vi "genIOL_Injection2.vi"(4 "Initial guess":dbl[](array[numeric])=[-67.99974822998047, 12.682350158691406, -0.8997803330421448, -0.012297453358769417], 6 "DH Params":cluster{"d_DH":dbl[][], "ty":dbl[][]}, 7 "endJ5":dbl=3200.0, 8 "OCT offset":dbl=11.0, 9 "endPt":dbl[](array[numeric])=[8.48840241312517, 12.608494085712664, 1.4642729158965477], 10 "PC path":path=path "D:/IRISSoft LV2016 beta/Host Demo/ThorlabsData/Eye1/VSCAN_0008.raw", 11 "Iris path":path=path "D:/IRISSoft LV2016 beta/Host Demo/ThorlabsData/Eye1/VSCAN_0007.raw") -> (0 "Whole_traj":dbl[][](array[numeric]), 1 "Inject_traj":dbl[][](array[numeric]))   [LabVIEW 2016]
uses:
  <vilib>/Math Plots/3D Math Plots/3D Scatter/3D Scatter XCtrl/3D Scatter.xctl
  <vilib>/Utility/file.llb/Read Delimited Spreadsheet (DBL).vi
  <vilib>/Utility/file.llb/Write Delimited Spreadsheet (DBL).vi
  <vilib>/Math Plots/3D Math Plots/3D Scatter/3D Scatter Datatype/Public/Plot Helper (Vector).vi
  <vilib>/Analysis/NI_AALBase.lvlib
  <vilib>/Analysis/1siggen.llb/Ramp Pattern by Samples.vi
  <vilib>/gmath/NI_Gmath.lvlib
  Subsystems/Global Variables.vi
  <vilib>/Math Plots/3D Math Plots/3D Scatter/3D Scatter Datatype/3D Scatter Datatype.lvclass
  <vilib>/Math Plots/3D Math Plots/3D Plot/3D Plot Datatype/3D Plot Datatype.lvclass
panel:
  in  "Theta":dbl
  out "Actual Injection Plot 2":refnum<class "3D Plot Datatype.lvclass">[](xcontrol)
  out "current loop # 2":dbl
  out "Actual joint angles":dbl[][](array[numeric])
  out "Planned joint angles":dbl[][](array[numeric])
  out "Planned injection":dbl[][](array[numeric])
  out "time":dbl[](array[numeric])
  out "Implement joint angles":dbl[][](graph)
  out "min dist":dbl
  out "Planed joint angles":dbl[][](graph)
  out "Actual joint angles":dbl[][](graph)
  out "traj":dbl[][](array[numeric])
  out "max dist":dbl
  out "Offset":dbl[][](array[numeric])
  out "Planed Injection Plot":refnum<class "3D Plot Datatype.lvclass">[](xcontrol)
  out "current loop #":dbl
  out "x coordinates size 3":dbl
  out "x coordinates size 2":dbl
  out "x coordinates size":dbl
  out "x coordinates":dbl[](array[numeric])
  out "z coordinates":dbl[](array[numeric]) format="%#_13g"
  out "y coordinates":dbl[](array[numeric]) format="%#_13g"
  out "x coodi 2nd":dbl[](array[numeric]) format="%#_13g"
  in  "Total Time":dbl=60.0
  in  "Arm ID Ind":i32
  in  "Tip out Posit":dbl[](array[numeric])=[0.0, 0.0, 0.0] caption="Position [mm]" format="%#.3f"
  out "zVisTraj":dbl[](array[numeric]) format="%_6g"
  out "yVisTraj":dbl[](array[numeric]) format="%_6g"
  out "xVisTraj":dbl[](array[numeric]) format="%_6g"
  in  "Sampling Rate [Hz]":i32=1000
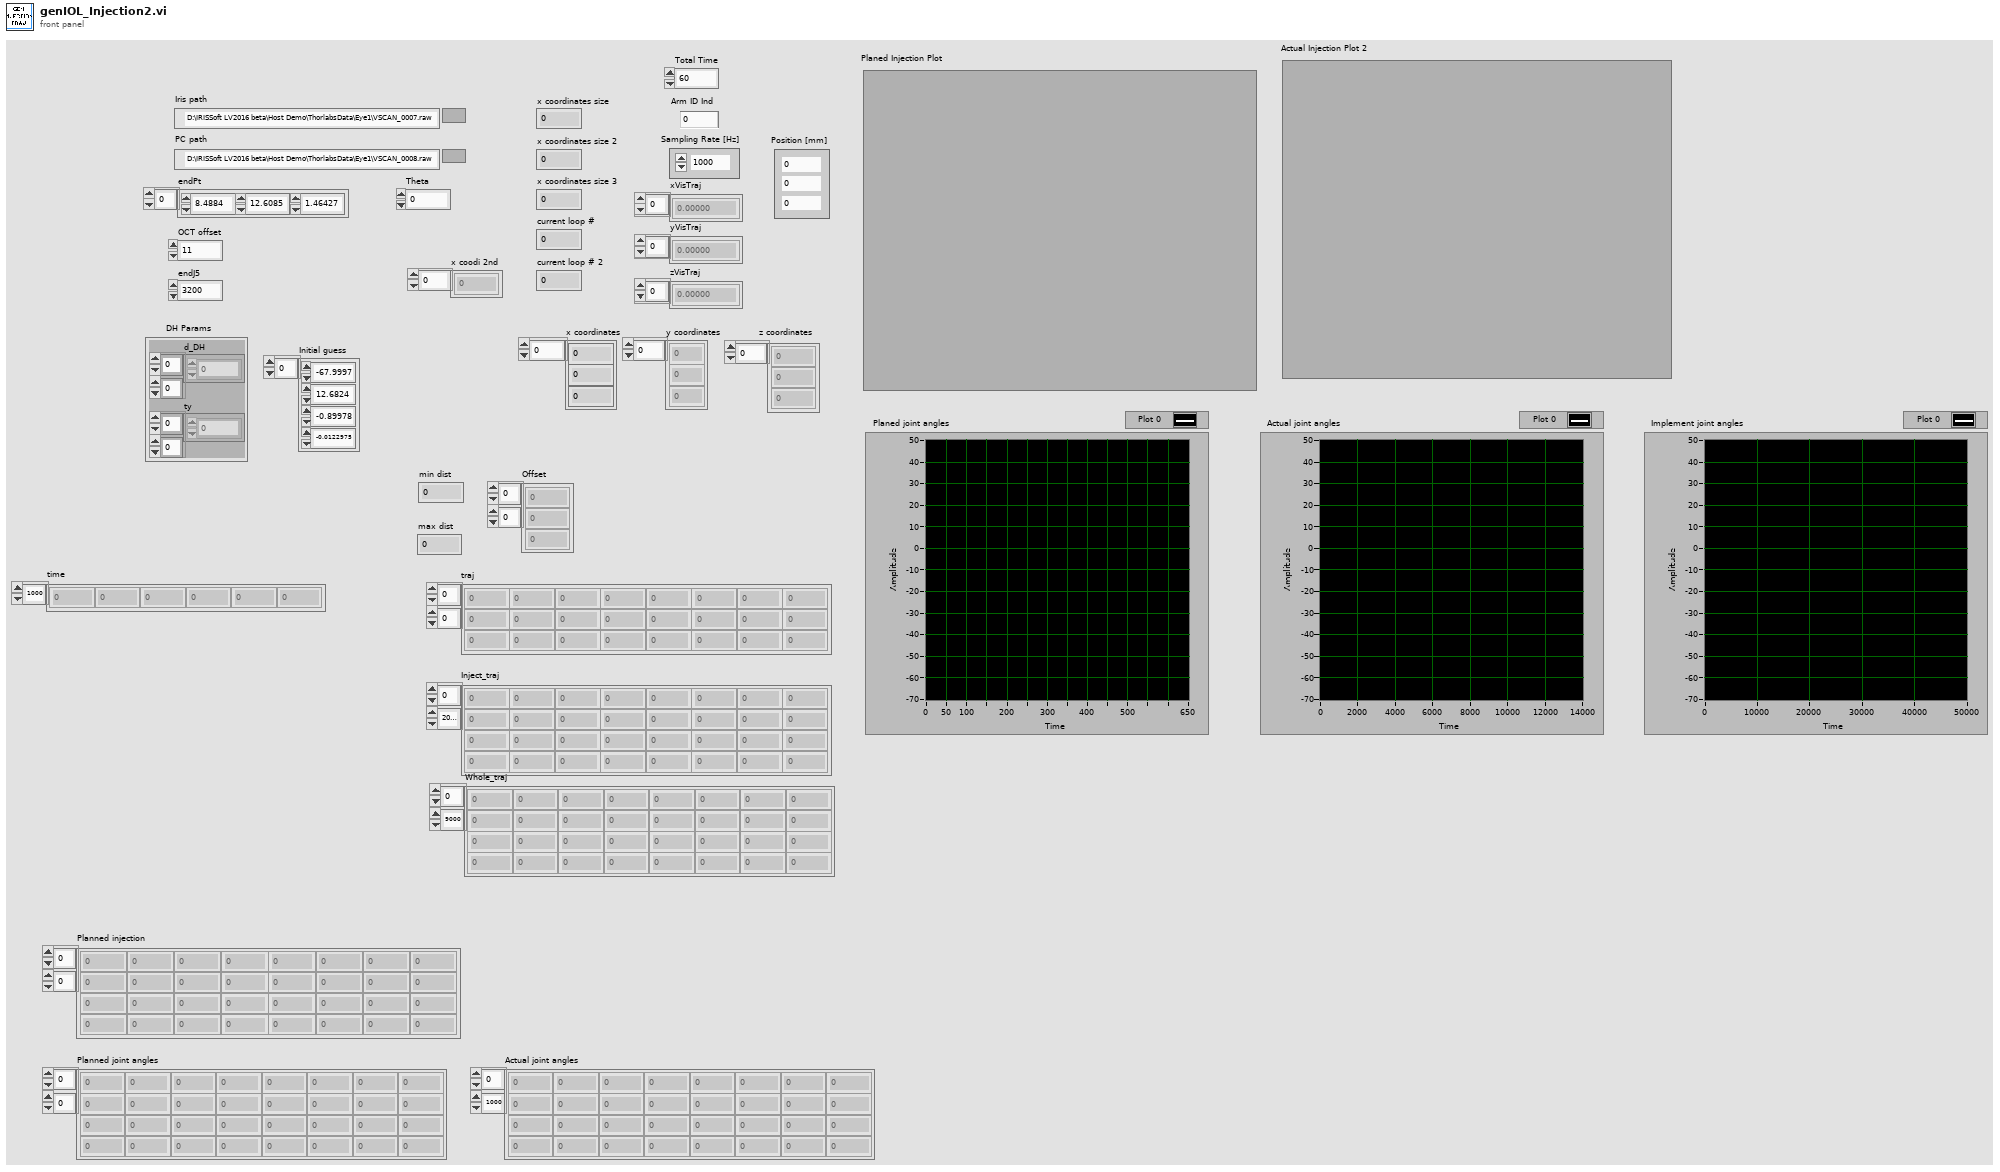
[diagram p1: front panel]
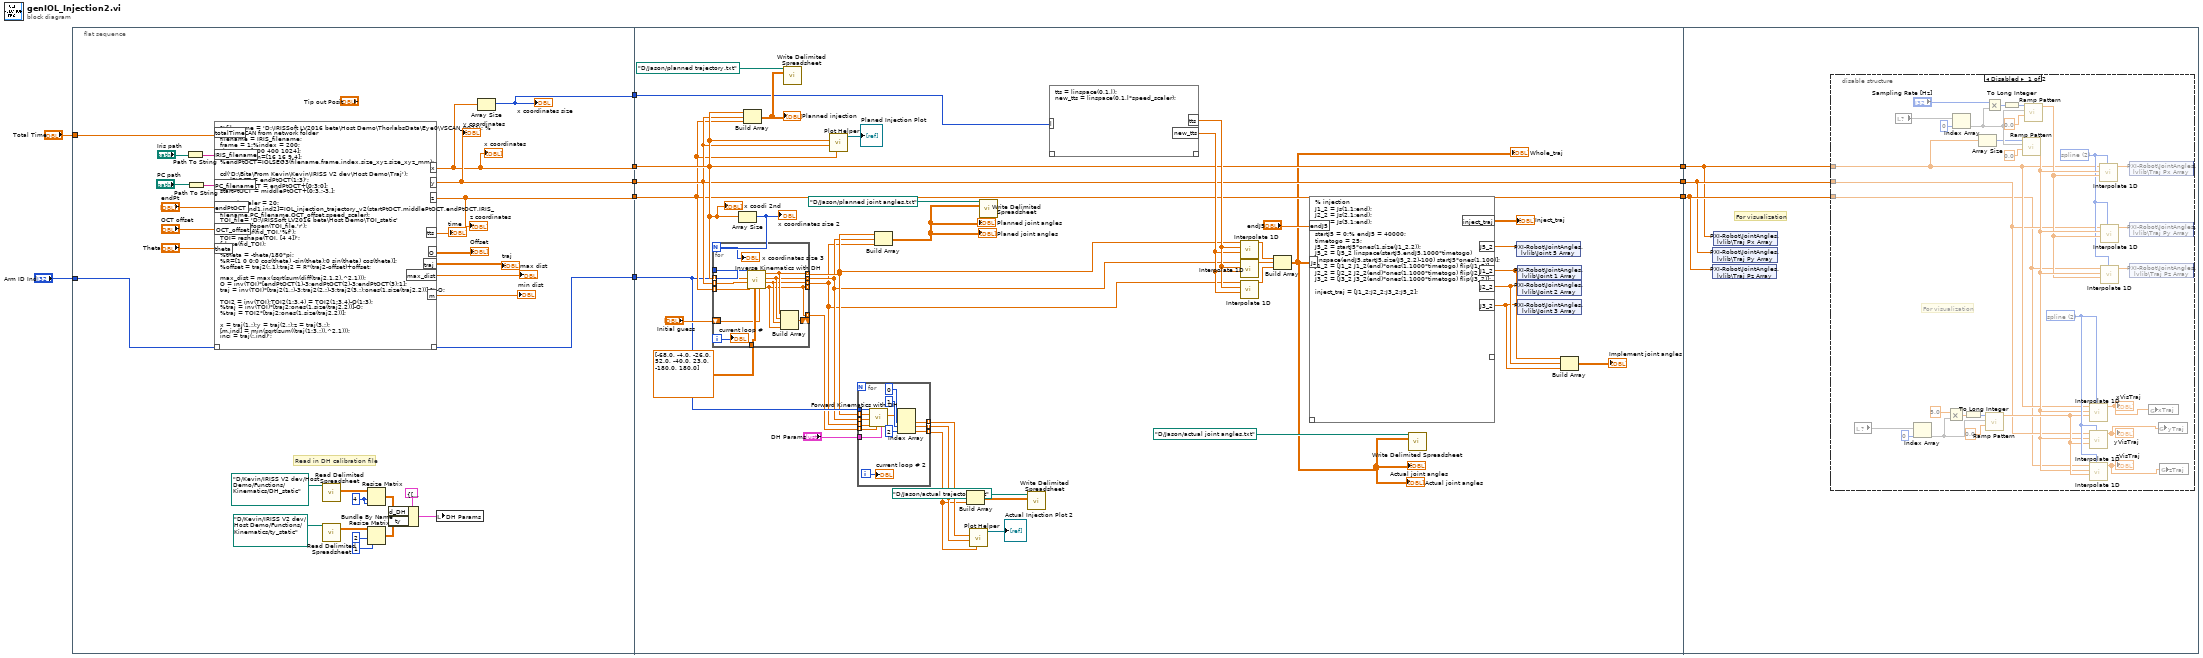
[diagram p0: block diagram]
diagram:
  n1 = flat-sequence {
    tunnel: "Arm ID Ind" -> [w12]
    tunnel: [w36] -> w6
    tunnel: [w38] -> w5
    tunnel: [w37] -> w4
    tunnel: "Total Time" -> [w39]
    tunnel: [w24] -> w2
    tunnel: [w12] -> w1
    tunnel: [w62] -> w9
    tunnel: [w61] -> w8
    tunnel: [w60] -> w7
    tunnel: w6 -> [w62]
    tunnel: w5 -> [w61]
    tunnel: w4 -> [w60]
    tunnel: w2 -> [w43]
    tunnel: w1 -> [w54]
    tunnel: w9 -> [w105]
    tunnel: w8 -> [w106]
    tunnel: w7 -> [w107]
    frame #0 {
      w21 = 4 ("number of rows")
      # "Read in DH calibration file"
      n2 = Path To String(path="Iris path") -> (string=w31:string)
      n3 = Path To String(path="PC path") -> (string=w32:string)
      n4 = script code="%filename = 'D:\\IRISSoft LV2016 beta\\Host Demo\\ThorlabsData\\Eye0\\VSCAN_0021'; % read VSCAN from network folder \nfilename = IRIS_filename;\nframe = 1;%index = 200;\nsize_xyz=[400 400 1024];\nsize_xyz_mm=[16 16 9.4];\n%endPtOCT=IOLSEG3(filename,frame,index,size_xyz,size_xyz_mm);\n\ncd('D:\\Bita\\From Kevin\\Kevin\\IRISS V2 dev\\Host Demo\\Traj');\nendPtOCT = endPtOCT(1:3)';\nmiddlePtOCT = endPtOCT+[0;3;0];\nstartPtOCT = middlePtOCT+[0;3.;-3.];\n\nspeed_scaler = 20;\n[tts,traj2,ind1,ind2]=IOL_injection_trajectory_v2(startPtOCT,middlePtOCT,endPtOCT,IRIS_filename,PC_filename,OCT_offset,speed_scaler);\nTOI_file= 'D:\\IRISSoft LV2016 beta\\Host Demo\\TOI_static'\nfid_TOI = fopen(TOI_file,'r');\nTOI=fscanf(fid_TOI,'%f');\nTOI= reshape(TOI, [4 4])';\nfclose(fid_TOI);\n\n%theta = -theta/180*pi;\n%R=[1 0 0;0 cos(theta) -sin(theta);0 sin(theta) cos(theta)];\n%offset = traj2(:,1);traj2 = R*(traj2-offset)+offset;\n\nmax_dist = max(sqrt(sum(diff(traj2,1,2).^2,1)));\nO = inv(TOI)*[endPtOCT(1)-3;endPtOCT(2)-3;endPtOCT(3);1];\ntraj = inv(TOI)*[traj2(1,:)-3;traj2(2,:)-3;traj2(3,:);ones(1,size(traj2,2))];%-O;\n\nTOI2 = inv(TOI);TOI2(1:3,4) = TOI2(1:3,4)-O(1:3);\n%traj = inv(TOI)*[traj2;ones(1,size(traj2,2))]-O;\n%traj = TOI2*[traj2;ones(1,size(traj2,2))];\n\nx = traj(1,:);y = traj(2,:);z = traj(3,:);\n[m,ind] = min(sqrt(sum((traj(1:3,:)).^2,1)));\ninci = traj(:,ind)';"("totalTime"=w39, "IRIS_filename"=w31, "PC_filename"=w32, "endPtOCT"="endPt", "OCT_offset"="OCT offset", "theta"="Theta") -> ("x"=w36:dbl[], "y"=w38:dbl[], "z"=w37:dbl[], "O"=→"Offset":dbl[][], "max_dist"=→"max dist":dbl, "traj"=→"traj":dbl[][], "m"=→"min dist":dbl, "tts"=→"time":dbl[])  [unwired: 1 in, 1 out]
      "y coordinates" <- w38
      "z coordinates" <- w37
      "x coordinates" <- w36
      n5 = call-poly <vilib>:"Read Delimited Spreadsheet.vi"("file path (dialog if empty)"=path "D:/Kevin/IRISS V2 dev/Host Demo/Functions/Kinematics/DH_static" ("file path (use dialog)")) -> ("all rows"=w22:dbl[][])  [unwired: 9 in, 5 out]
      n6 = call-poly <vilib>:"Read Delimited Spreadsheet.vi"("file path (dialog if empty)"=path "D:/Kevin/IRISS V2 dev/Host Demo/Functions/Kinematics/ty_static" ("file path (use dialog)")) -> ("all rows"=w20:dbl[][])  [unwired: 9 in, 5 out]
      n7 = Resize Matrix(1:w21, 2:w21, 4:w22) -> (0:w16:dbl[][])
      n8 = Resize Matrix(1:1 ("number of columns"), 2:2 ("number of rows"), 4:w20) -> (0:w15:dbl[][])
      n9 = Bundle By Name(cluster=cluster{"d_DH":dbl[][], "ty":dbl[][]} {"d_DH"=[[0.0, -0.04858099004841317, 1.1971672750675049, 0.0], [0.0, -1.576475511297109, 0.0, 0.0], [-0.3552491783526254, 0.0, -1.1064589410656984, 0.2058446720735121], [-1.0573457532495087, 1.0278049025155533, 0.011917110633363169, -0.004023577880993236]], "ty"=[[0.04320445582455471], [0.011728642746432275]]} ("input cluster"), "d_DH"=w16, "ty"=w15) -> (w13:cluster{"d_DH":dbl[][], "ty":dbl[][]})
      n10 = local write "DH Params"(w13) -> ()
      n11 = Array Size(array=w36) -> (size(s)=w24:i32)
      "x coordinates size" <- w24
    }
    frame #1 {
      n12 = Array Size(array=w62) -> (size(s)=w77:i32)
      "x coordinates size 2" <- w77
      n13 = for {
        N: w77 -> [w104]
        tunnel: w54 -> [w101]
        tunnel: w62 -> [w100] mode=indexing
        tunnel: w61 -> [w99] mode=indexing
        tunnel: w60 -> [w98] mode=indexing
        tunnel: [w94] -> w47 mode=indexing
        tunnel: [w95] -> w48 mode=indexing
        tunnel: [w93] -> w46 mode=indexing
        tunnel: dbl[][] [[-68.0, -4.0], [-26.0, 52.0], [-40.0, 23.0], [-180.0, 180.0]] ("Joint Limits") -> [w97]
        shift-right: [w102] -> _
        shift-left: "Initial guess" -> [w96]
        tunnel: [w92] -> _ mode=indexing
        tunnel: [w92] -> w40 mode=indexing
        i -> [w103]
        n14 = call "Inverse Kinematics with DH.vi"("Initial guess"=w96, "Joint Limits"=w97, "armID"=w101, "z"=w98, "y"=w99, "x"=w100) -> ("j4"=w92:dbl, "j3"=w93:dbl, "j2"=w94:dbl, "j1"=w95:dbl)  [unwired: 2 in]
        n15 = Build Array(w95, w94, w93, w92) -> (w102:dbl[])
        "x coordinates size 3" <- w104
        "current loop #" <- w103
      }
      n16 = Build Array(w62, w61, w60) -> (w59:dbl[][])
      "Planned injection" <- w59
      n17 = call-poly <vilib>:"Write Delimited Spreadsheet.vi"("file path (dialog if empty)"=path "D:/Jason/planned trajectory.txt", "2D data"=w59) -> ()  [unwired: 12 in, 2 out]
      n18 = call-poly <vilib>:"Plot Helper.vi"("z vector"=w60, "y vector"=w61, "x vector"=w62) -> ("3D Plot lvclass Array out"=→"Planed Injection Plot":refnum<class "3D Plot Datatype.lvclass">[])  [unwired: 3 in, 5 out]
      n19 = for {
        tunnel: w54 -> [w84]
        tunnel: w48 -> [w85] mode=indexing
        tunnel: w47 -> [w83] mode=indexing
        tunnel: w46 -> [w82] mode=indexing
        tunnel: [w88] -> w53 mode=indexing
        tunnel: [w87] -> w52 mode=indexing
        tunnel: [w86] -> w51 mode=indexing
        tunnel: "DH Params" -> [w80]
        tunnel: w40 -> [w78] mode=indexing
        i -> [w79]
        n20 = call "Forward Kinematics with DH.vi"("DH Params"=w80, "j4"=w78, "j3"=w82, "j2"=w83, "j1"=w85, "armID"=w84) -> ("XYZ With DH Calibration"=w81:dbl[])  [unwired: 3 in, 2 out]
        n21 = Index Array(array=w81, index #1=0 ("index"), index #2=1 ("index"), index #3=2 ("index")) -> (element #1=w88:dbl, element #2=w87:dbl, element #3=w86:dbl)
        "current loop # 2" <- w79
      }
      n22 = Build Array(w48, w47, w46) -> (w57:dbl[][])
      "Planed joint angles" <- w57
      "Planned joint angles" <- w57
      n23 = Build Array(w53, w52, w51) -> (w50:dbl[][])
      n24 = call-poly <vilib>:"Plot Helper.vi"("z vector"=w51, "y vector"=w52, "x vector"=w53) -> ("3D Plot lvclass Array out"=→"Actual Injection Plot 2":refnum<class "3D Plot Datatype.lvclass">[])  [unwired: 3 in, 5 out]
      n25 = call-poly <vilib>:"Write Delimited Spreadsheet.vi"("file path (dialog if empty)"=path "D:/Jason/planned joint angles.txt", "2D data"=w57) -> ()  [unwired: 12 in, 2 out]
      n26 = call-poly <vilib>:"Write Delimited Spreadsheet.vi"("file path (dialog if empty)"=path "D:/Jason/actual trajectory2.txt", "2D data"=w50) -> ()  [unwired: 12 in, 2 out]
      n27 = script code="tts = linspace(0,1,l);\nnew_tts = linspace(0,1,l*speed_scaler);"("l"=w43) -> ("new_tts"=w73:dbl[], "tts"=w74:dbl[])  [unwired: 1 in, 1 out]
      n28 = call <vilib>:"Interpolate 1D.vi"("xi"=w73, "X"=w74, "Y"=w48) -> ("yi"=w72:dbl[])  [unwired: 6 in, 2 out]
      n29 = call <vilib>:"Interpolate 1D.vi"("xi"=w73, "X"=w74, "Y"=w47) -> ("yi"=w71:dbl[])  [unwired: 6 in, 2 out]
      n30 = call <vilib>:"Interpolate 1D.vi"("xi"=w73, "X"=w74, "Y"=w46) -> ("yi"=w70:dbl[])  [unwired: 6 in, 2 out]
      n31 = Build Array(w72, w71, w70) -> (w42:dbl[][])
      "Actual joint angles" <- w42
      "Whole_traj" <- w42
      "Actual joint angles" <- w42
      n32 = script code="% injection\nJ1_2 = Js(1,1:end);\nJ2_2 = Js(2,1:end);\nJ3_2 = Js(3,1:end);\n\nstartJ5 = 0;% endJ5 = 40000;\ntimetogo = 25;\nJ5_2 = startJ5*ones(1,size(J1_2,2));\nJ5_2 = [J5_2 linspace(startJ5,endJ5,1000*timetogo) linspace(endJ5,startJ5,size(J5_2,2)-100) startJ5*ones(1,100)];\nJ1_2 = [J1_2 J1_2(end)*ones(1,1000*timetogo) flip(J1_2)];\nJ2_2 = [J2_2 J2_2(end)*ones(1,1000*timetogo) flip(J2_2)];\nJ3_2 = [J3_2 J3_2(end)*ones(1,1000*timetogo) flip(J3_2)];\n\ninject_traj = [J1_2;J2_2;J3_2;J5_2];"("Js"=w42, "endJ5"="endJ5") -> ("J1_2"=w67:dbl[], "J2_2"=w66:dbl[], "J3_2"=w65:dbl[], "J5_2"=w68:dbl[], "inject_traj"=→"Inject_traj":dbl[][])  [unwired: 1 in, 1 out]
      n33 = call-poly <vilib>:"Write Delimited Spreadsheet.vi"("file path (dialog if empty)"=path "D:/Jason/actual joint angles.txt", "2D data"=w42) -> ()  [unwired: 12 in, 2 out]
      n34 = shared-variable "PXI-Robot\\JointAngles.lvlib\\Joint 5 Array"(w68) -> ()  [unwired: 1 in, 1 out]
      n35 = shared-variable "PXI-Robot\\JointAngles.lvlib\\Joint 1 Array"(w67) -> ()  [unwired: 1 in, 1 out]
      n36 = shared-variable "PXI-Robot\\JointAngles.lvlib\\Joint 2 Array"(w66) -> ()  [unwired: 1 in, 1 out]
      n37 = shared-variable "PXI-Robot\\JointAngles.lvlib\\Joint 3 Array"(w65) -> ()  [unwired: 1 in, 1 out]
      n38 = Build Array(w67, w66, w65) -> (→"Implement joint angles":dbl[][])
      "x coodi 2nd" <- w62
    }
    frame #2 {
      # "For visualization"
      n39 = shared-variable "PXI-Robot\\JointAngles.lvlib\\Traj Py Array"(w106) -> ()  [unwired: 1 in, 1 out]
      n40 = shared-variable "PXI-Robot\\JointAngles.lvlib\\Traj Pz Array"(w107) -> ()  [unwired: 1 in, 1 out]
      n41 = shared-variable "PXI-Robot\\JointAngles.lvlib\\Traj Px Array"(w105) -> ()  [unwired: 1 in, 1 out]
      n42 = disable-structure shown="Disabled" {
        disable-tunnel: w105 -> [w113 _]
        disable-tunnel: w106 -> [w112 _]
        disable-tunnel: w107 -> [w111 _]
        frame Disabled {
          w125 = 2 items=["nearest", "linear", "spline", "cubic Hermite", "Lagrange"] ("method")
          w114 = 2 items=["nearest", "linear", "spline", "cubic Hermite", "Lagrange"] ("method")
          # "For visualization"
          n43 = local read item#-1() -> (w119)
          n44 = local read item#-1() -> (w137)
          n45 = Index Array(array=w119, index=0) -> (element=w120)
          n46 = Multiply(x=5.0, y=w120) -> (x*y=w122:dbl)
          n47 = Index Array(array=w137, index=0) -> (element=w130)
          n48 = To Long Integer(number=w122) -> (32bit integer=w123:i32)
          n49 = Array Size(array=w113) -> (size(s)=w129:i32)
          n50 = call-poly <vilib>:"Ramp Pattern.vi"("start"=0.0, "end"=w120, "samples"=w123) -> ("Ramp Pattern"=w117:dbl[])  [unwired: 7 in, 1 out]
          n51 = Multiply(x="Sampling Rate [Hz]", y=w130) -> (x*y=w133:i32)
          n52 = To Long Integer(number=w133) -> (32bit integer=w134:i32)
          n53 = call-poly <vilib>:"Ramp Pattern.vi"("start"=0.0, "end"=w130, "samples"=w129) -> ("Ramp Pattern"=w116:dbl[])  [unwired: 7 in, 1 out]
          n54 = call-poly <vilib>:"Ramp Pattern.vi"("start"=0.0, "end"=w130, "samples"=w134) -> ("Ramp Pattern"=w115:dbl[])  [unwired: 7 in, 1 out]
          n55 = call <vilib>:"Interpolate 1D.vi"("method"=w125, "xi"=w117, "X"=w116, "Y"=w113) -> ("yi"=w108:dbl[])  [unwired: 5 in, 2 out]
          "xVisTraj" <- w108
          n56 = call <vilib>:"Interpolate 1D.vi"("method"=w125, "xi"=w117, "X"=w116, "Y"=w112) -> ("yi"=w109:dbl[])  [unwired: 5 in, 2 out]
          "yVisTraj" <- w109
          n57 = call <vilib>:"Interpolate 1D.vi"("method"=w125, "xi"=w117, "X"=w116, "Y"=w111) -> ("yi"=w110:dbl[])  [unwired: 5 in, 2 out]
          "zVisTraj" <- w110
          n58 = call <vilib>:"Interpolate 1D.vi"("method"=w114, "xi"=w115, "X"=w116, "Y"=w113) -> ("yi"=w127:dbl[])  [unwired: 5 in, 2 out]
          n59 = call <vilib>:"Interpolate 1D.vi"("method"=w114, "xi"=w115, "X"=w116, "Y"=w112) -> ("yi"=w128:dbl[])  [unwired: 5 in, 2 out]
          n60 = call <vilib>:"Interpolate 1D.vi"("method"=w114, "xi"=w115, "X"=w116, "Y"=w111) -> ("yi"=w126:dbl[])  [unwired: 5 in, 2 out]
          n61 = shared-variable "PXI-Robot\\JointAngles.lvlib\\Traj Px Array"(w127) -> ()  [unwired: 1 in, 1 out]
          n62 = shared-variable "PXI-Robot\\JointAngles.lvlib\\Traj Py Array"(w128) -> ()  [unwired: 1 in, 1 out]
          n63 = shared-variable "PXI-Robot\\JointAngles.lvlib\\Traj Pz Array"(w126) -> ()  [unwired: 1 in, 1 out]
          n64 = global write "Global Variables.vi" "xTraj"(w108) -> ()
          n65 = global write "Global Variables.vi" "yTraj"(w109) -> ()
          n66 = global write "Global Variables.vi" "zTraj"(w110) -> ()
        }
        frame Enabled {
        }
      }
    }
  }
